vi "cb_SPIEngine.vi"() -> ()   [LabVIEW 2014]
uses:
  Program Files (x86)/National Instruments/LabVIEW 2014/user.lib/_NI SPI IP/FPGA/Controllers/Public/Spi Master Inputs.ctl
  Program Files (x86)/National Instruments/LabVIEW 2014/user.lib/_NI SPI IP/FPGA/Controllers/Public/Spi Master Outputs.ctl
  Program Files (x86)/National Instruments/LabVIEW 2014/user.lib/_NI SPI IP/FPGA/Controllers/Public/Transfer Settings.ctl
panel:
  out "Read Data":u64
  out "Read Data Valid?":bool
  in  "start":bool=TRUE
  out "IP Strobe Count":u64
  out "API Strobe Count":u64
  in  "SPI PHY Settings":T1={"Divide Value"=20, "Transfer Length (bits)"=32, "CS Asserted Polarity"=TRUE, "Clock Polarity (CPOL)"=TRUE, "Clock Phase (CPHA)"=FALSE, "Lengthen MISO Setup"=FALSE, "Direction Change Bit"=0, "MOSI Starts as Output"=FALSE, "Tristatable MOSI"=FALSE} {"Direction Change Bit" max=64 step=1; "Transfer Length (bits)" min=1 max=64 step=1}
  in  "stop":bool
  out "spi output":T2
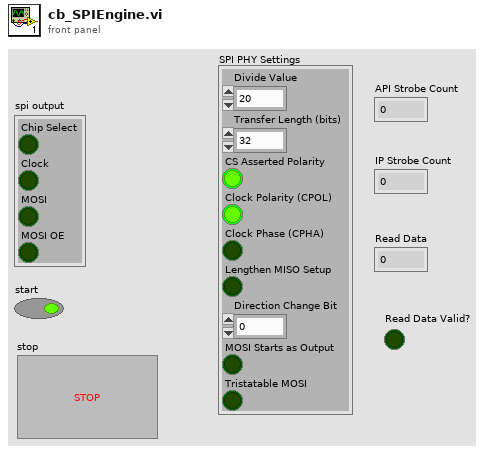
[diagram p1: front panel]
types:
  T1 = typedef "NI SPI IP (FPGA).lvlib/Transfer Settings.ctl" = cluster{"Divide Value":u8, "Transfer Length (bits)":u8, "CS Asserted Polarity":bool, "Clock Polarity (CPOL)":bool, "Clock Phase (CPHA)":bool, "Lengthen MISO Setup":bool, "Direction Change Bit":u8, "MOSI Starts as Output":bool, "Tristatable MOSI":bool}
  T2 = typedef "NI SPI IP (FPGA).lvlib/Spi Master Outputs.ctl" = cluster{"Chip Select":bool, "Clock":bool, "MOSI":bool, "MOSI OE":bool}
  T3 = typedef "Internal Data (SPI API).ctl" = cluster{"DLU To SPI Engine Data FIFO":refnum<k21>, "SPI Engine to DLU Data FIFO":refnum<k21>, "Data to SPI Engine (Cache) Register":refnum<k21>, "SPI PHY Settings to SPI Engine (Cahche) Register":refnum<k21>}
  T4 = typedef "NI SPI IP (FPGA).lvlib/Spi Master Inputs.ctl" = cluster{"MISO":bool}
  T5 = typedef "SPI Transaction Packet.ctl" = cluster{"Chip Select ID":u8, "SPI Data":u64, "Start Strobe":bool, "SPI PHY Settings":cluster{"Divide Value":u8, "Transfer Length (bits)":u8, "CS Asserted Polarity":bool, "Clock Polarity (CPOL)":bool, "Clock Phase (CPHA)":bool, "Lengthen MISO Setup":bool, "Direction Change Bit":u8, "MOSI Starts as Output":bool, "Tristatable MOSI":bool}}
  T6 = typedef "SPI Response Information.ctl" = cluster{"Data to Node":u64, "Node Id":u16}
  T7 = typedef "NI SPI IP FPGA.lvlib/Spi Master Outputs.ctl" = cluster{"Chip Select":bool, "Clock":bool, "MOSI":bool, "MOSI OE":bool}
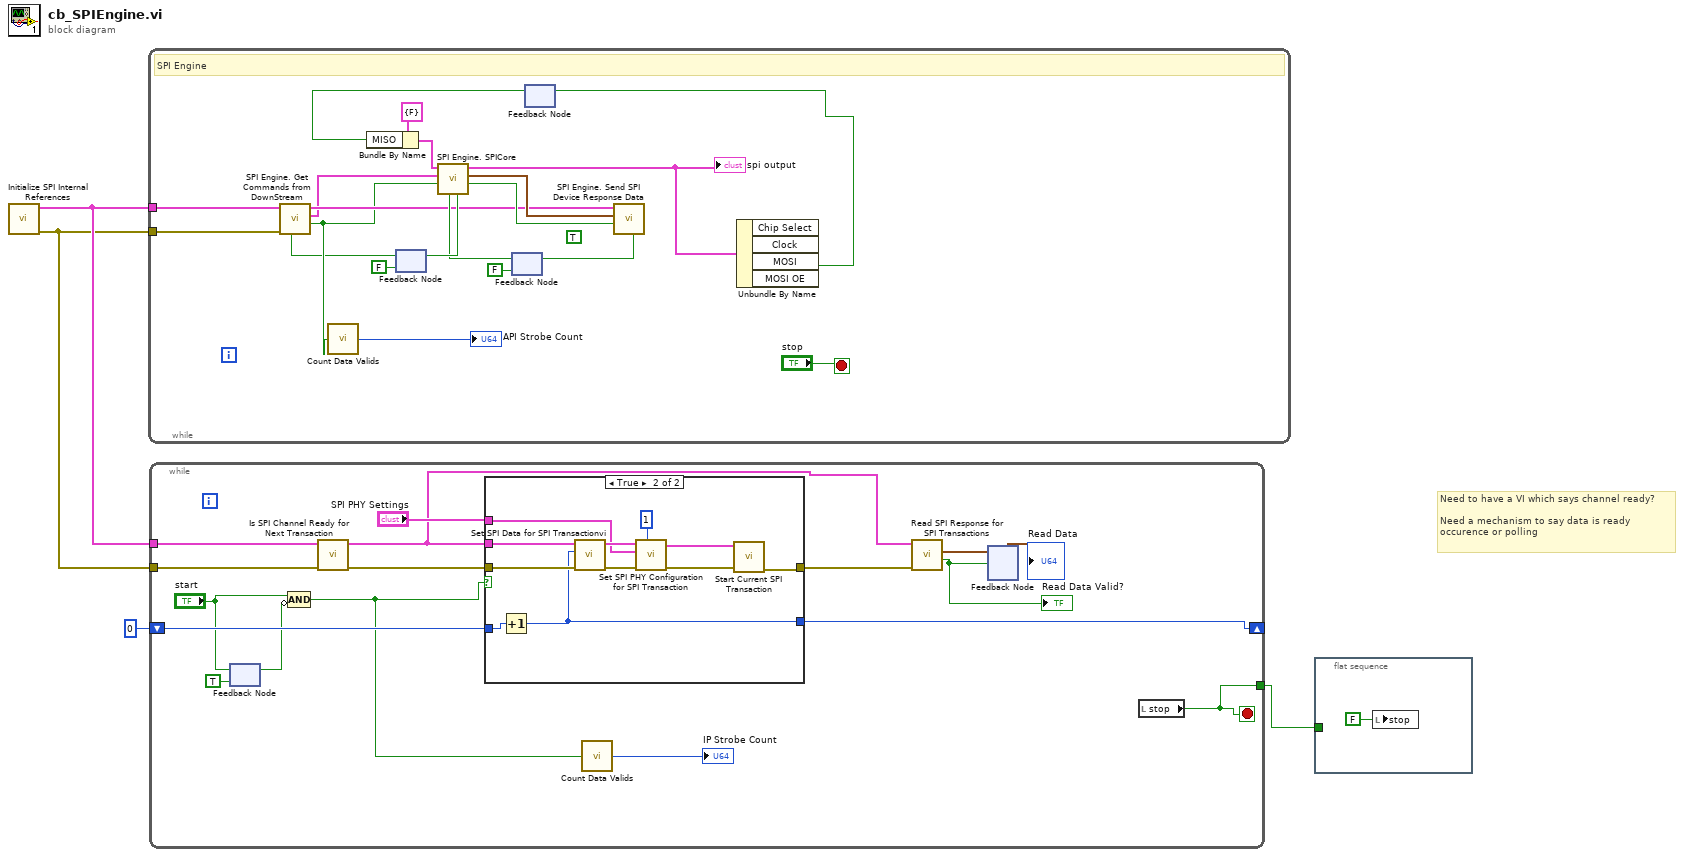
[diagram p0: block diagram]
diagram:
  # "Need to have a VI which says channel ready?\n\nNeed a mechanism to say data is ready\noccurence or polling"
  n1 = call "Initialize SPI Internal References.vi"() -> ("error out"=w2:errorcluster, "SPI API References"=w4:T3)  [unwired: 10 in]
  n2 = while {
    tunnel: w4 -> [w16]
    tunnel: w2 -> [w13]
    stop <- "stop" stop-if-true
    (unwired) TRUE
    # "SPI Engine"
    n3 = feedback #1(FALSE ("ready for input")) -> (w10:bool)
    n4 = call "SPI Engine. Get Commands from DownStream.vi"("Ready for Output"=w10, "error in"=w13, "Private Data In"=w16) -> ("Output Valid"=w11:bool, "SPI Transaction Packet"=w12:T5, "Private Data Out"=w14:T3)  [unwired: 4 in, 2 out]
    n5 = call "Count Data Valids.vi"("Data Valid"=w11) -> ("Counter"=→"API Strobe Count":u64)  [unwired: 14 in]
    n6 = feedback #2(FALSE ("Ready for Input")) -> (w19:bool)
    n7 = feedback #3() -> (w6:bool)  [unwired: 1 in]
    n8 = Bundle By Name(cluster=T4 {"MISO"=FALSE} ("SPI DIO Input"), "MISO"=w6) -> (w5:T4)
    n9 = call "SPI Engine. SPICore.vi"("Ready for Output"=w19, "Input Valid"=w11, "SPI Information In"=w12, "SPI DIO Input"=w5) -> ("Output Valid"=w21:bool, "SPI Output Data"=w22:T6, "SPI DIO Output"=w9:T7, "Ready For Input"=w24:bool)  [unwired: 3 in, 1 out]
    "spi output" <- w9
    n10 = feedback-in #1(w24) -> ()
    n11 = call "SPI Engine. Send SPI Device Response Data.vi"("Input Valid"=w21, "Input Data"=w22, "Private Data In"=w14) -> ("Ready for Input"=w20:bool)  [unwired: 5 in, 3 out]
    n12 = feedback-in #2(w20) -> ()
    n13 = Unbundle By Name(w9) -> ("MOSI"=w7:bool)  [unwired: 3 out]
    n14 = feedback-in #3(w7) -> ()
  }
  n15 = while {
    tunnel: w4 -> [w39]
    tunnel: [w38] -> w3
    tunnel: w2 -> [w37]
    shift-right: [w34] -> _
    shift-left: u8 0 -> [w35]
    stop <- w38 stop-if-true
    n16 = feedback-in #4("start") -> ()
    n17 = feedback #4(TRUE ("start")) -> (w31:bool)
    n18 = Compound Arithmetic op=AND("start", invert w31) -> (w29:bool)
    n19 = call "Is SPI Channel Ready for Next Transaction.vi"("error in"=w37, "Private Data In"=w39) -> ("error out"=w36:errorcluster, "Private Data Out"=w25:T3)  [unwired: 6 in, 2 out]
    n20 = case shown="True" w29 {
      tunnel: w25 -> [_ w53]
      tunnel: "SPI PHY Settings" -> [_ w50]
      tunnel: [_ w45] -> w33
      tunnel: w36 -> [_ w48]
      tunnel: w35 -> [w42 w47]
      tunnel: [w42 w46] -> w34
      frame False {
      }
      frame True {
        n21 = Increment(x=w47) -> (x+1=w46:u8)
        n22 = call "Set SPI Data for SPI Transactionvi.vi"("error in"=w48, "Data In"=w46, "Private Data In"=w53) -> ("error out"=w51:errorcluster, "Private Data Out"=w52:T3)  [unwired: 7 in]
        n23 = call "Set SPI PHY Configuration for SPI Transaction.vi"("Chip Select"=u8 1, "error in"=w51, "SPI PHY Settings"=w50, "Private Data In"=w52) -> ("error out"=w43:errorcluster, "Private Data Out"=w44:T3)  [unwired: 6 in]
        n24 = call "Start Current SPI Transaction.vi"("error in"=w43, "Private Data In"=w44) -> ("error out"=w45:errorcluster)  [unwired: 7 in, 2 out]
      }
    }
    n25 = call "Count Data Valids.vi"("Data Valid"=w29) -> ("Counter"=→"IP Strobe Count":u64)  [unwired: 14 in]
    n26 = call "Read SPI Response for SPI Transactions.vi"("error in"=w33, "Private Data In"=w25) -> ("Read Data Valid?"=w28:bool, "Read Data"=w27:T6)  [unwired: 6 in, 2 out]
    "Read Data Valid?" <- w28
    n27 = feedback-in #5(w27, w28) -> ()
    n28 = feedback #5() -> (→"Read Data":T6)  [unwired: 1 in]
    n29 = local read "stop"() -> (w38:bool)
  }
  n30 = flat-sequence {
    tunnel: w3 -> [_]
    frame #0 {
      n31 = local write "stop"(FALSE ("stop")) -> ()
    }
  }
